vi "Estructura_datos.vi"() -> ()   [LabVIEW 2020]
panel:
  out "Numeric":i32
  out "Slide 2":dbl(slide) scale=0.0..10.0
  in  "Slide":dbl(slide) scale=0.0..10.0
  # "Panel Frontal"
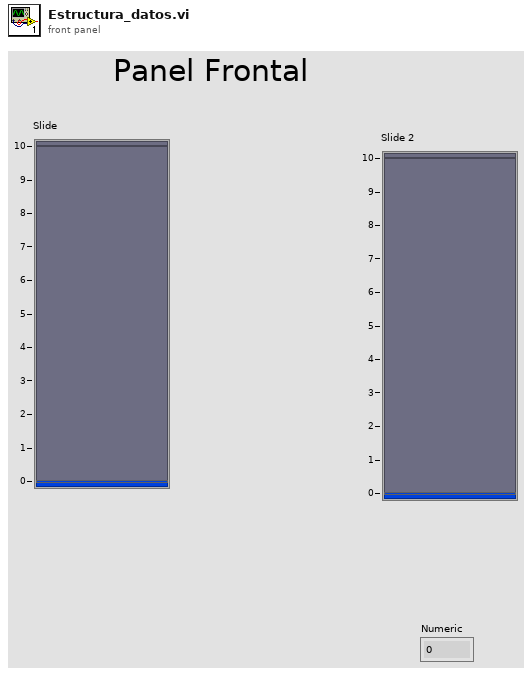
[diagram p1: front panel]
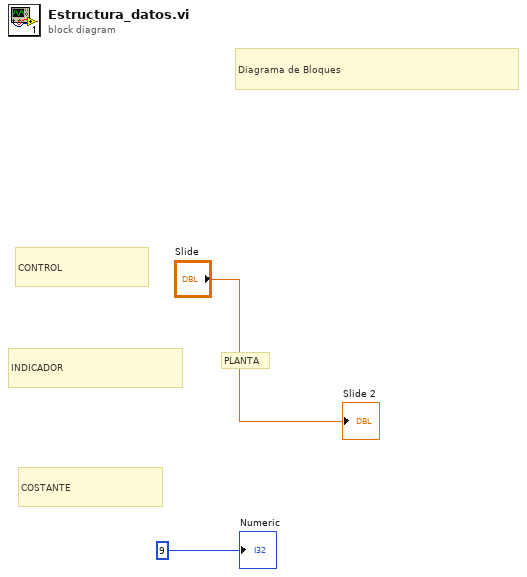
[diagram p0: block diagram]
diagram:
  # "PLANTA"
  # "COSTANTE"
  # "INDICADOR"
  # "CONTROL"
  # "Diagrama de Bloques"
  "Slide 2" <- "Slide"
  "Numeric" <- 9
